vi "Drive Motor Control.vi"(11 "Drive Reference In":T1={"RobotDriveDevRef"={"DevStatus"={"status"=FALSE, "code"=0, "source"=""}, "Motors[]"=[], "Square Inputs"=FALSE, "Max Output"=1.0}, "Drive PTO Solenoid"={"DevStatus"={"status"=FALSE, "code"=0, "source"=""}, "Pneumatics Control Module"=0, "Forward Solenoid Channel"=enum."Invalid", "Reverse Solenoid Channel"=enum."Invalid"}, "High Gear Solenoid"={"DevStatus"={"status"=FALSE, "code"=0, "source"=""}, "Pneumatics Control Module"=0, "Forward Solenoid Channel"=enum."Invalid", "Reverse Solenoid Channel"=enum."Invalid"}}) -> (3 "Drive Reference Out":T1={"RobotDriveDevRef"={"DevStatus"={"status"=FALSE, "code"=0, "source"=""}, "Motors[]"=[], "Square Inputs"=FALSE, "Max Output"=1.0}, "Drive PTO Solenoid"={"DevStatus"={"status"=FALSE, "code"=0, "source"=""}, "Pneumatics Control Module"=0, "Forward Solenoid Channel"=enum."Invalid", "Reverse Solenoid Channel"=enum."Invalid"}, "High Gear Solenoid"={"DevStatus"={"status"=FALSE, "code"=0, "source"=""}, "Pneumatics Control Module"=0, "Forward Solenoid Channel"=enum."Invalid", "Reverse Solenoid Channel"=enum."Invalid"}})   [LabVIEW 2016]
uses:
  Drive Reference.ctl
  <vilib>/Rock Robotics/WPI/RobotDrive/WPI_RobotDriveDevRef.ctl
  <vilib>/Rock Robotics/WPI/MotorControl/WPI_MotorControlDeviceRef.ctl
  <vilib>/Rock Robotics/WPI/MotorControl/WPI_MotorControlType.ctl
  <vilib>/Rock Robotics/SystemInterfaces/DIO/FPGA_DIOPWMChannel.ctl
  <vilib>/Rock Robotics/WPI/PWM/WPI_PWMDeadband.ctl
  <vilib>/Rock Robotics/WPI/Solenoid/WPI_SolenoidDevRef.ctl
  <vilib>/Rock Robotics/WPI/Solenoid/WPI_SolenoidChannel.ctl
  <vilib>/Rock Robotics/WPI/Solenoid/WPI_SolenoidValue.ctl
  Robot Values.vi
  <vilib>/Rock Robotics/WPI/Solenoid/WPI_SolenoidSetEnum.vi
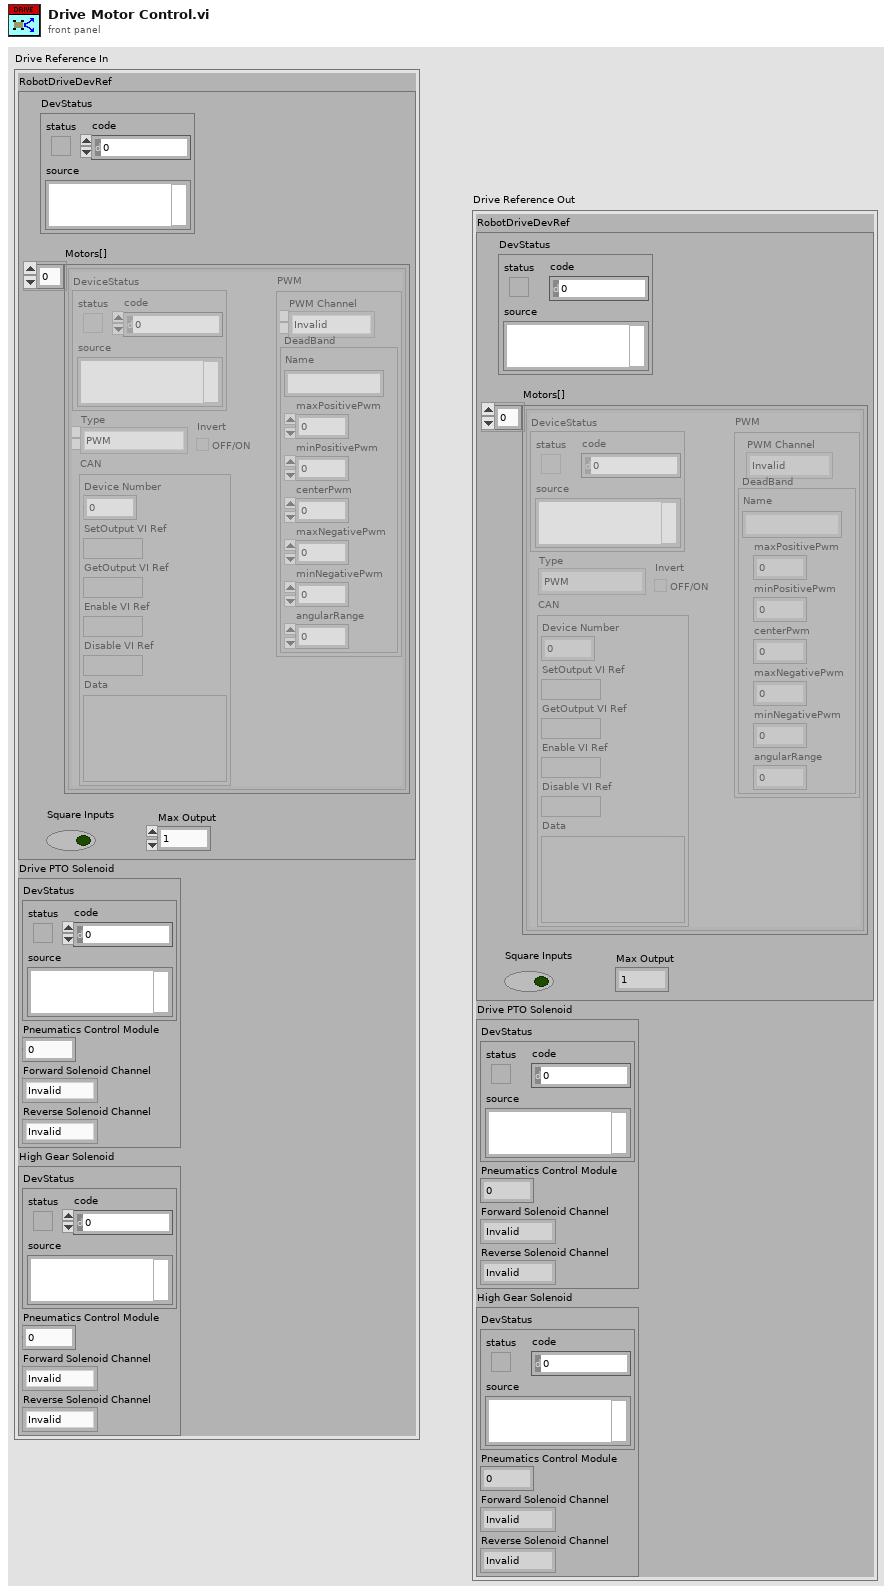
[diagram p1: front panel]
types:
  T1 = typedef "Drive Reference.ctl" = cluster{"RobotDriveDevRef":T2, "Drive PTO Solenoid":T7, "High Gear Solenoid":T7}
  T2 = typedef "WPI_RobotDriveDevRef.ctl" = cluster{"DevStatus":errorcluster, "Motors[]":T3[], "Square Inputs":bool, "Max Output":dbl}
  T3 = typedef "WPI_MotorControlDeviceRef.ctl" = cluster{"DeviceStatus":errorcluster, "Type":T4, "PWM":cluster{"PWM Channel":T5, "DeadBand":T6}, "CAN":cluster{"Device Number":u8, "SetOutput VI Ref":variant, "GetOutput VI Ref":variant, "Enable VI Ref":variant, "Disable VI Ref":variant, "Data":variant}, "Invert":bool}
  T4 = typedef "WPI_MotorControlType.ctl" = enum16{"PWM", "CAN"}
  T5 = typedef "FPGA_DIOPWMChannel.ctl" = enum8{"PWM 0", "PWM 1", "PWM 2", "PWM 3", "PWM 4", "PWM 5", "PWM 6", "PWM 7", "PWM 8", "PWM 9", "PWM MXP 0", "PWM MXP 1", "PWM MXP 2", "PWM MXP 3", "PWM MXP 4", "PWM MXP 5", "PWM MXP 6", "PWM MXP 7", "PWM MXP 8", "PWM MXP 9", "Invalid"}
  T6 = typedef "WPI_PWMDeadband.ctl" = cluster{"Name":string, "maxPositivePwm":i32, "minPositivePwm":i32, "centerPwm":i32, "maxNegativePwm":i32, "minNegativePwm":i32, "angularRange":u16}
  T7 = typedef "WPI_SolenoidDevRef.ctl" = cluster{"DevStatus":errorcluster, "Pneumatics Control Module":u8, "Forward Solenoid Channel":T8, "Reverse Solenoid Channel":T8}
  T8 = typedef "WPI_SolenoidChannel.ctl" = enum8{"Solenoid 0", "Solenoid 1", "Solenoid 2", "Solenoid 3", "Solenoid 4", "Solenoid 5", "Solenoid 6", "Solenoid 7", "Invalid"}
  T9 = typedef "WPI_SolenoidValue.ctl" = enum16{"Off", "On", "Forward", "Reverse"}
  T10 = typedef "Robot Values.ctl" = cluster{"Robot Drive":cluster{"Left Motor Power":dbl, "Right Motor Power":dbl, "Left Encoder Value":dbl, "Right Encoder Value":dbl, "High Gear?":bool, "PTO?":bool}, "Sensors":cluster{"Gyro Angle":u16, "Recalibrate Gyro":bool, "Reset Gyro":bool, "Ultrasonic":dbl}, "Shooter":cluster{"Prep Wheels":bool, "Shoot":bool, "Left Shooter Wheel Speed":dbl, "Wheels Moving":bool, "Shooter Prepped":bool, "Shooter RPS SP":dbl, "Shooting?":bool, "Left Shooter Wheel Power":dbl, "Right Shooter Wheel Power":dbl, "Acquisition Conveyor Power":dbl, "Hopper Beater Bar Power":dbl, "Filtered Left Shooter Speed":dbl, "Acquisition Motor Power":dbl, "Joystick Add":dbl}, "Robot States":cluster{"Drive mode":string, "Alliance":T11, "Position":T12}, "Gear":cluster{"Ejection Active":bool}}
  T11 = typedef "WPI_DriverStationAllianceInfo.ctl" = enum16{"Red", "Blue", "Invalid"}
  T12 = typedef "WPI_DriverStationPositionInfo.ctl" = enum16{"1", "2", "3"}
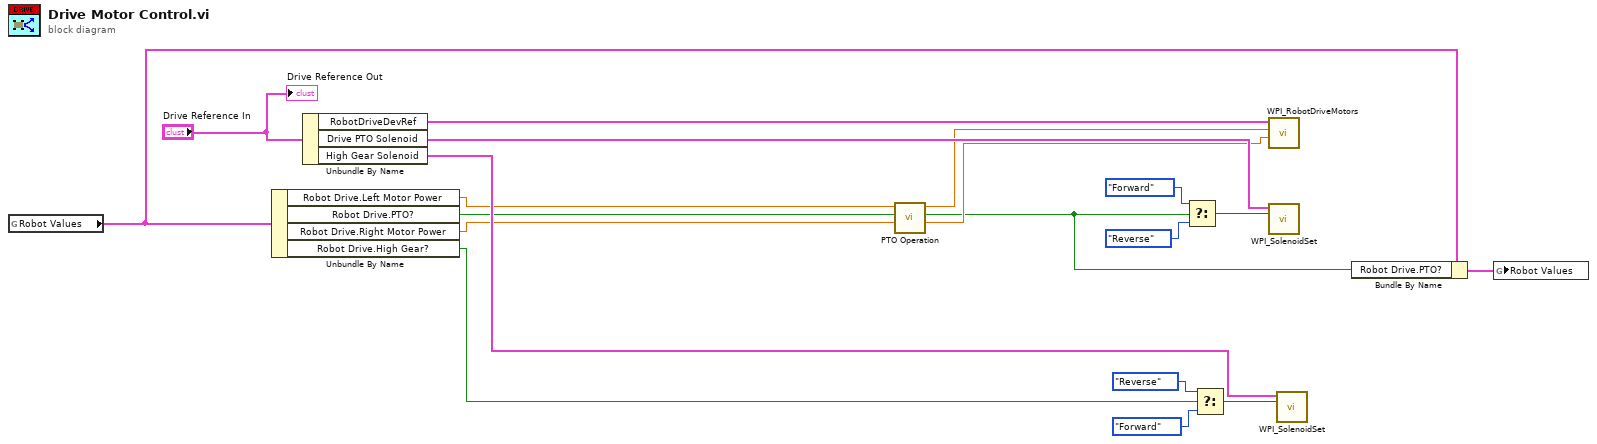
[diagram p0: block diagram]
diagram:
  n1 = global read "Robot Values.vi" "Robot Values"() -> (w3:T10)
  n2 = Unbundle By Name(w3) -> ("Robot Drive.Left Motor Power"=w7:dbl, "Robot Drive.PTO?"=w8:bool, "Robot Drive.Right Motor Power"=w6:dbl, "Robot Drive.High Gear?"=w9:bool)
  n3 = Unbundle By Name("Drive Reference In") -> ("RobotDriveDevRef"=w19:T2, "Drive PTO Solenoid"=w16:T7, "High Gear Solenoid"=w10:T7)
  n4 = call "PTO Operation.vi"("Left Motor Power In"=w7, "PTO  Engaged IN?"=w8, "Right Motor Power In"=w6) -> ("Left Motor Power Out"=w5:dbl, "PTO Engaged? Out"=w1:bool, "Right Motor Power Out"=w4:dbl)  [unwired: 5 in]
  n5 = Select(t=WPI_SolenoidValue."Forward", s=w1, f=WPI_SolenoidValue."Reverse" ("Value")) -> (s? t:f=w17:T9)
  n6 = Select(t=WPI_SolenoidValue."Reverse", s=w9, f=WPI_SolenoidValue."Forward" ("Value")) -> (s? t:f=w13:T9)
  n7 = call <vilib>:"WPI_RobotDriveMotors.vi"("RightSpeed"=w4, "LeftSpeed"=w5, "RobotDriveDevRef"=w19) -> ()  [unwired: 6 in, 3 out]
  n8 = call-poly <vilib>:"WPI_SolenoidSet.vi"("Value"=w17, "SolenoidDevRef"=w16) -> ()  [unwired: 8 in, 2 out]
  n9 = call-poly <vilib>:"WPI_SolenoidSet.vi"("Value"=w13, "SolenoidDevRef"=w10) -> ()  [unwired: 8 in, 2 out]
  n10 = Bundle By Name(cluster=w3, "Robot Drive.PTO?"=w1) -> (w2:T10)
  n11 = global write "Robot Values.vi" "Robot Values"(w2) -> ()
  "Drive Reference Out" <- "Drive Reference In"
